vi "MListbox Get One Row.vi"(8 "error in (no error)":errorcluster, 10 "index (row)":i32, 11 "Multicolumn ListBox in":refnum<class "Multicolumn ListBox.lvclass">) -> (0 "error out":errorcluster, 2 "Array":string[](array[string]), 3 "Multicolumn ListBox out":refnum<class "Multicolumn ListBox.lvclass">)   [LabVIEW 2018, in "Multicolumn ListBox.lvclass"]
uses:
  Multicolumn ListBox.lvclass
  Multicolumn ListBox.lvclass/Multicolumn ListBox.ctl
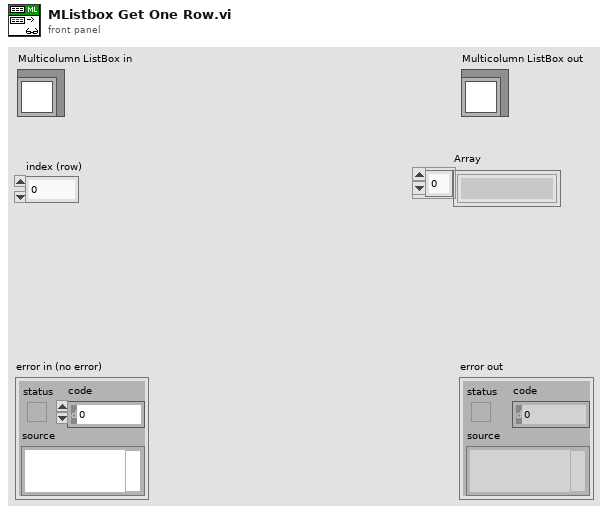
[diagram p1: front panel]
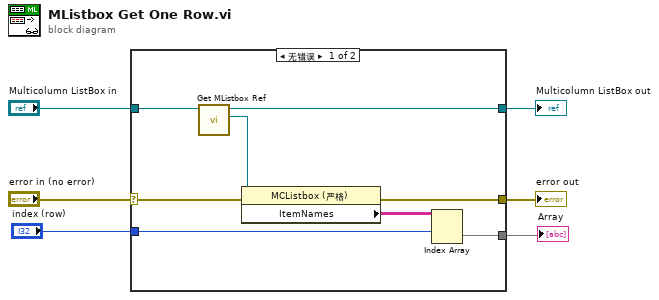
[diagram p0: block diagram]
diagram:
  n1 = case shown="无错误" "error in (no error)" {
    selector: "error in (no error)" -> [w8 w16]
    tunnel: [w7 w16] -> w5
    tunnel: [w13 w15] -> w3
    tunnel: "Multicolumn ListBox in" -> [w14 w15]
    tunnel: "index (row)" -> [w10 _]
    tunnel: [w9 _] -> w1
    frame No Error {
      n2 = call "Get MListbox Ref.vi"("Multicolumn ListBox in"=w14) -> ("MListbox Ref"=w12:refnum<vi>, "Multicolumn ListBox out"=w13:refnum<class "Multicolumn ListBox.lvclass">)  [unwired: 8 in, 1 out]
      n3 = property class="MCListbox (严格)"(reference=w12, error in=w8) -> (error out=w7:errorcluster, "ItemNames"=w11:string[][])  [unwired: 1 out]
      n4 = Index Array(array=w11, index (row)=w10) -> (element=w9:string[])  [unwired: 1 in]
    }
    frame Error {
    }
  }
  "error out" <- w5
  "Multicolumn ListBox out" <- w3
  "Array" <- w1
